vi "Update Lua Palettes.vi"() -> ()   [LabVIEW 2020, in "Lua DevUtil.lvlib"]
uses:
  Lua DevUtil.lvlib
  <vilib>/Palette API/Palette Menu/Public Type Define/Palette Data.ctl
  <vilib>/Palette API/Palette Menu/Public Type Define/View Format.ctl
  <vilib>/Palette API/Palette Menu/Public Type Define/Items.ctl
  <vilib>/Palette API/Palette Menu/Public Type Define/Item.ctl
  <vilib>/Palette API/Palette Menu/Public Type Define/Help Info.ctl
  <vilib>/Palette API/Palette Menu/Public Type Define/Synchronize Info.ctl
  <vilib>/Utility/miscctls.llb/LVMapReplaceAction.ctl
  <vilib>/Palette API/Palette Menu/Public Type Define/Palette type.ctl
  85e9b90b-9151-4f09-9030-f452b0e3cf19.vi
  <vilib>/Comparison/Less/Less Functor/Less Functor.lvclass
  <vilib>/Palette API/Palette Menu/Palette Menu.lvlib
panel:
  out "errors":T1(array[cluster])
  out "Lua menus":T2(c390)
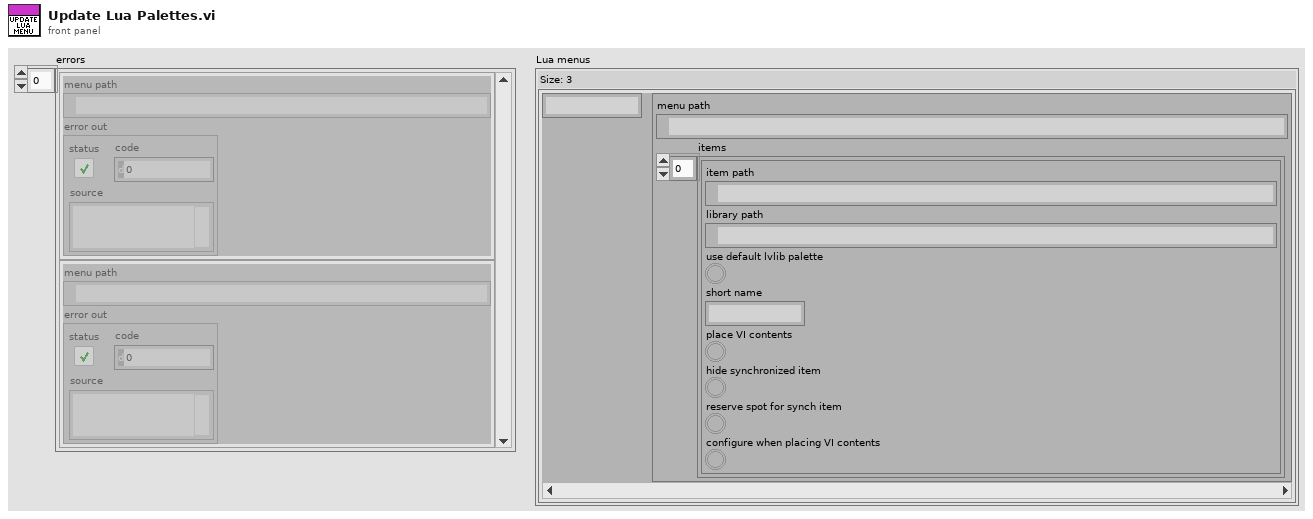
[diagram p1: front panel]
types:
  T1 = cluster{"menu path":path, "error out":errorcluster}[]
  T2 = map{string, cluster{"menu path":path, "items":cluster{"item path":path, "library path":path, "use default lvlib palette":bool, "short name":string, "place VI contents":bool, "hide synchronized item":bool, "reserve spot for synch item":bool, "configure when placing VI contents":bool}[]}}
  T3 = cluster{"item path":path, "library path":path, "use default lvlib palette":bool, "short name":string, "place VI contents":bool, "hide synchronized item":bool, "reserve spot for synch item":bool, "configure when placing VI contents":bool}
  T4 = typedef "LVMapReplaceAction.ctl" = enum32{"Modify Entry only if found", "Add or Modify Entry", "Delete Entry"}
  T5 = cluster{"menu path":path, "items":cluster{"item path":path, "library path":path, "use default lvlib palette":bool, "short name":string, "place VI contents":bool, "hide synchronized item":bool, "reserve spot for synch item":bool, "configure when placing VI contents":bool}[]}
  T6 = cluster{"item path":path, "library path":path, "use default lvlib palette":bool, "short name":string, "place VI contents":bool, "hide synchronized item":bool, "reserve spot for synch item":bool, "configure when placing VI contents":bool}[]
  T7 = typedef "Palette Menu.lvlib/View Format.ctl" = u16
  T8 = typedef "Palette Menu.lvlib/Palette Data.ctl" = cluster{"display name":string, "view format":T7, "palette width":i16, "items":T9, "256 color icon":picture, "B&W color icon":picture, "help information":T11, "palette description":string, "synchronize information":T12}
  T9 = typedef "Palette Menu.lvlib/Items.ctl" = T10[]
  T10 = typedef "Palette Menu.lvlib/Item.ctl" = cluster{"item path":path, "library path":path, "use default lvlib palette":bool, "short name":string, "place VI contents":bool, "hide synchronized item":bool, "reserve spot for synch item":bool, "configure when placing VI contents":bool}
  T11 = typedef "Palette Menu.lvlib/Help Info.ctl" = cluster{"help tag":string, "help file path ":path}
  T12 = typedef "Palette Menu.lvlib/Synchronize Info.ctl" = cluster{"synchronize with directory":bool, "synchronize directory path":path}
  T13 = typedef "Palette Menu.lvlib/Palette type.ctl" = i32
  T14 = cluster{"menu path":path, "error out":errorcluster}
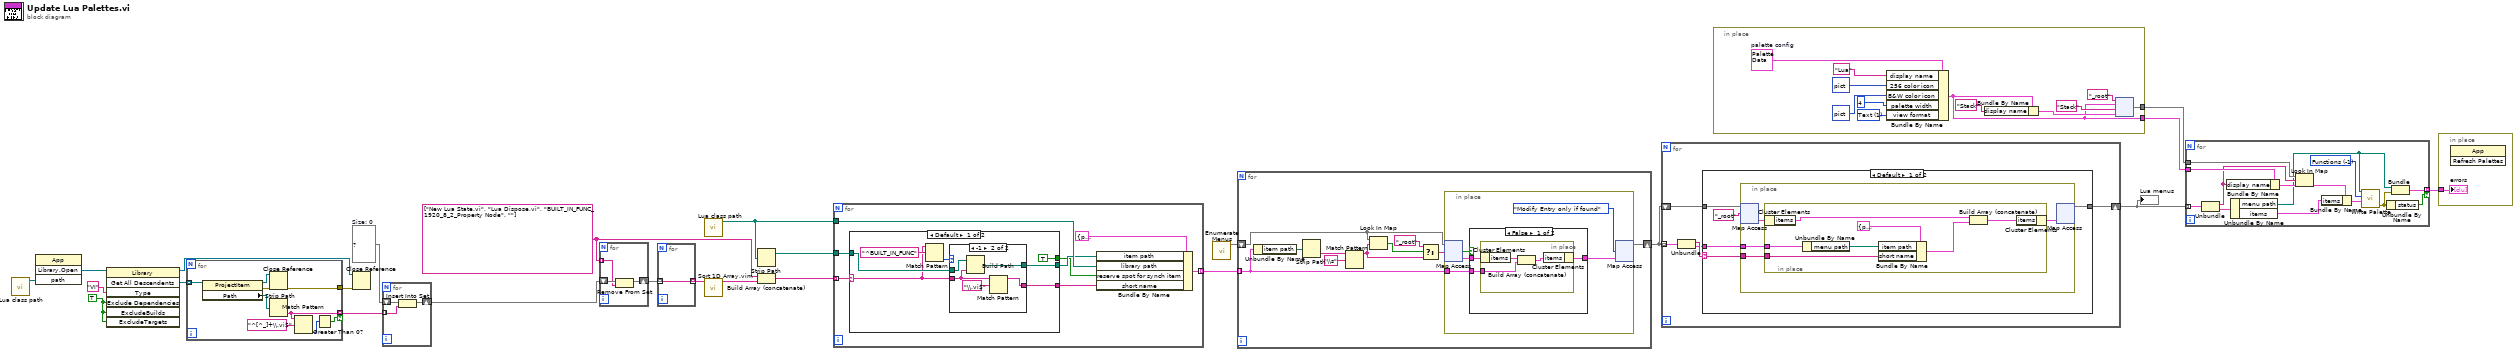
[diagram p0: block diagram]
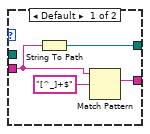
[diagram p4: hidden frame]
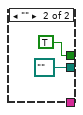
[diagram p5: hidden frame]
diagram:
  w15 = set{string} {}  # Size: 0
  w20 = TRUE ("ExcludeDependencies")
  w1 = string[] ["New Lua State.vi", "Lua Dispose.vi", "BUILT_IN_FUNC_1920_8_2_Property Node", ""]
  n1 = call "Lua class path.vi"() -> ("palette file path"=w23:path)  [unwired: 11 in]
  n2 = invoke class="App" method="Library.Open"("path"=w23) -> ("Open Library"=w22:refnum<vi>)  [unwired: 3 in, 3 out]
  n3 = invoke class="Library" method="Get All Descendents"(reference=w22, "Type"="VI", "Exclude Dependencies"=w20, "ExcludeBuilds"=w20, "ExcludeTargets"=w20) -> (reference out=w18:refnum<vi>, "All Descendents"=w19:refnum<vi>[])  [unwired: 2 in, 5 out]
  n4 = for {
    tunnel: w19 -> [w33] mode=indexing
    tunnel: [w25] -> w16 mode=indexing if=w27
    tunnel: [w30] -> w17
    n5 = property class="ProjectItem"(reference=w33) -> (reference out=w31:refnum<vi>, error out=w32:errorcluster, "Path"=w26:path)  [unwired: 1 in]
    n6 = Close Reference(reference=w31, error in (no error)=w32) -> (error out=w30:errorcluster)
    n7 = Strip Path(path=w26) -> (name=w25:string)  [unwired: 1 out]
    n8 = Match Pattern(string=w25, regular expression="^[^_]+\\.vi$") -> (offset past match=w28:i32)  [unwired: 1 in, 3 out]
    n9 = Greater Than 0?(x=w28) -> (x > 0?=w27:bool)
  }
  n10 = Close Reference(reference=w18, error in (no error)=w17) -> ()  [unwired: 1 out]
  n11 = for {
    shift-right: [w36] -> w14
    shift-left: w15 -> [w34]
    tunnel: w16 -> [w35] mode=indexing
    n12 = Insert Into Set(10:w35, 11:w34) -> (3:w36:set{string})  [unwired: 1 out]
  }
  n13 = for {
    shift-right: [w38] -> w13
    shift-left: w14 -> [w39]
    tunnel: w1 -> [w37] mode=indexing
    n14 = Remove From Set(10:w37, 11:w39) -> (3:w38:set{string})  [unwired: 1 out]
  }
  n15 = for {
    tunnel: w13 -> [w40] mode=indexing
    tunnel: [w40] -> w12 mode=indexing
  }
  n16 = call "Lua class path.vi"() -> ("palette file path"=w24:path)  [unwired: 11 in]
  n17 = call "Sort 1D Array.vim"("unsorted array"=w12) -> ("sorted array"=w11:string[])  [unwired: 10 in]
  n18 = Strip Path(path=w24) -> (stripped path=w9:path)  [unwired: 1 out]
  n19 = Build Array (concatenate)(w1, w11) -> (w10:string[])
  n20 = for {
    tunnel: w10 -> [w46] mode=indexing
    tunnel: [w47] -> w7 mode=indexing
    tunnel: w24 -> [w45]
    tunnel: w9 -> [w44]
    n21 = case shown="Default" w46 {
      selector: w46 -> [w52 _]
      tunnel: w44 -> [w55 _]
      tunnel: [w51 path "" ("appended path")] -> w43
      tunnel: [w50 _] -> w42
      tunnel: [TRUE ("use default lvlib palette") TRUE ("use default lvlib palette")] -> w41
      frame Default {
        n22 = Match Pattern(string=w52, regular expression="^BUILT_IN_FUNC") -> (offset past match=w53:i32)  [unwired: 1 in, 3 out]
        n23 = case shown="-1" w53 {
          tunnel: w55 -> [_ w64]
          tunnel: w52 -> [w58 w62]
          tunnel: [w59 w63] -> w51
          tunnel: [w56 w60] -> w50
          frame Default {
            n24 = String To Path(string=w58) -> (path=w59:path)
            n25 = Match Pattern(string=w58, regular expression="[^_]+$") -> (match substring=w56:string)  [unwired: 1 in, 3 out]
          }
          frame -1 {
            n26 = Build Path(base path=w64, name or relative path=w62) -> (appended path=w63:path)
            n27 = Match Pattern(string=w62, regular expression="\\.vi$") -> (before substring=w60:string)  [unwired: 1 in, 3 out]
          }
        }
      }
      frame "" {
      }
    }
    n28 = Bundle By Name(cluster=T3 {"item path"=path "", "library path"=path "", "use default lvlib palette"=FALSE, "short name"="", "place VI contents"=FALSE, "hide synchronized item"=FALSE, "reserve spot for synch item"=TRUE, "configure when placing VI contents"=FALSE}, "item path"=w43, "library path"=w45, "reserve spot for synch item"=w41, "short name"=w42) -> (w47:T3)
  }
  n29 = call "Enumerate Menus.vi"() -> ("Lua menus"=w8:T2)  [unwired: 11 in]
  n30 = for {
    shift-right: [w73] -> w6
    shift-left: w8 -> [w71]
    tunnel: w7 -> [w72] mode=indexing
    n31 = Unbundle By Name(w72) -> ("item path"=w76:path)
    n32 = Strip Path(path=w76) -> (name=w75:string)  [unwired: 1 out]
    n33 = Match Pattern(string=w75, regular expression="\\s") -> (before substring=w69:string)  [unwired: 1 in, 3 out]
    n34 = Look In Map(map=w71, key=w69) -> (key not found?=w70:bool)  [unwired: 1 in, 1 out]
    n35 = Select(t="_root" ("regular expression"), s=w70, f=w69) -> (s? t:f=w67:string)
    n36 = in-place {
      in-place-border: w72 -> [w77]
      n37 = in-place-map #1(w71, w67) -> (w79:T5, w81:bool)  [unwired: 1 in]
      n38 = case shown="False" w81 {
        tunnel: [w82 w88] -> w80
        tunnel: w79 -> [w84 w88]
        tunnel: w77 -> [w83 _]
        frame False {
          n39 = in-place {
            in-place-border: w83 -> [w86]
            n40 = in-place-cluster #2(w84) -> ("items"=w87:T6)
            n41 = Build Array (concatenate)(w87, w86) -> (w85:T6)
            n42 = in-place-cluster #2("items"=w85) -> (w82:T5)
          }
        }
        frame True {
        }
      }
      n43 = in-place-map #1(w80, LVMapReplaceAction."Modify Entry only if found" ("action")) -> (w73:T2)  [unwired: 2 out]
    }
  }
  n44 = for {
    tunnel: w6 -> [w93] mode=indexing
    shift-right: [w90] -> w5
    shift-left: w6 -> [w91]
    n45 = Unbundle(w93) -> ("submatch 1"=w92:string, w89:T5)
    n46 = case shown="Default" w92 {
      selector: w92 -> [w95 _]
      tunnel: w91 -> [w98 w110]
      tunnel: [w96 w110] -> w90
      tunnel: w89 -> [w97 _]
      frame Default {
        n47 = in-place {
          in-place-border: w97 -> [w101]
          in-place-border: w95 -> [w99]
          n48 = in-place-map #3(w98, "_root") -> (w102:T5)  [unwired: 1 in, 1 out]
          n49 = in-place {
            in-place-border: w101 -> [w109]
            in-place-border: w99 -> [w104]
            n50 = in-place-cluster #4(w102) -> ("items"=w108:T6)
            n51 = Unbundle By Name(w109) -> ("menu path"=w105:path)
            n52 = Bundle By Name(cluster=T3 {"item path"=path "", "library path"=path "", "use default lvlib palette"=FALSE, "short name"="", "place VI contents"=FALSE, "hide synchronized item"=FALSE, "reserve spot for synch item"=FALSE, "configure when placing VI contents"=FALSE}, "item path"=w105, "short name"=w104) -> (w103:T3)
            n53 = Build Array (concatenate)(w108, w103) -> (w107:T6)
            n54 = in-place-cluster #4("items"=w107) -> (w100:T5)
          }
          n55 = in-place-map #3(w100) -> (w96:T2)  [unwired: 1 in, 2 out]
        }
      }
      frame "_root" {
      }
    }
  }
  "Lua menus" <- w5
  n56 = in-place {
    in-place-border: [w113] -> w4
    in-place-border: [w112] -> w3
    w111 = T7 1 items=["Icons", "Text", "Icons and Text"] ("view format")
    w122 = T8 {"display name"="Lua", "view format"=0, "palette width"=2, "items"=[], "256 color icon"=bytes[1182], "B&W color icon"=bytes[286], "help information"={"help tag"="", "help file path "=path ""}, "palette description"="", "synchronize information"={"synchronize with directory"=FALSE, "synchronize directory path"=path ""}}  # palette config
    n57 = Bundle By Name(cluster=w122, "display name"="Lua", "256 color icon"=picture bytes[1182], "B&W color icon"=picture bytes[286], "palette width"=i16 4, "view format"=w111) -> (w112:T8)
    n58 = Bundle By Name(cluster=w112, "display name"="Stack") -> (w114:T8)
    n59 = node("_root" ("key"), w112, "Stack" ("key"), w114) -> (w113:map{string, T8})
  }
  n60 = for {
    tunnel: w5 -> [w136] mode=indexing
    tunnel: w4 -> [w135]
    tunnel: w3 -> [w134]
    tunnel: [w126] -> w2 mode=indexing if=w125
    w130 = T13 -1 items=["Functions"=-1, "Controls"=-2] ("palette type")
    n61 = Unbundle(w136) -> ("submatch 1"=w132:string, w131:T5)
    n62 = Bundle By Name(cluster=w134, "display name"=w132) -> (w133:T8)
    n63 = Unbundle By Name(w131) -> ("menu path"=w127:path, "items"=w128:T6)
    n64 = Look In Map(map=w135, key=w132, default value=w133) -> (value=w129:T8)  [unwired: 1 out]
    n65 = Bundle By Name(cluster=w129, "items"=w128) -> (w124:T8)
    n66 = call <vilib>:"Write Palette.vi"("palette data"=w124, "palette type"=w130, "palette path"=w127) -> ("error out"=w123:errorcluster)  [unwired: 8 in]
    n67 = Unbundle By Name(w123) -> ("status"=w125:bool)
    n68 = Bundle("menu path"=w127, "error out"=w123) -> (w126:T14)  [unwired: 1 in]
  }
  n69 = in-place {
    in-place-border: w2 -> [w137]
    n70 = invoke class="App" method="Refresh Palettes"() -> ()  [unwired: 3 in, 3 out]
    "errors" <- w137
  }
